vi "Set VI Reentrant Setting.vi"() -> ()   [LabVIEW 2016]
doc: "A wrapper engine for setting re-entrant setting for all VIs in a folder."
uses:
  <vilib>/Utility/error.llb/DialogType.ctl
  SLL Queued State Machine/Queue Driver/Create Queue.vi
  SLL Queued State Machine/Queue Driver/Enqueue an Item to Queue.vi
  SLL Queued State Machine/Queue Driver/Dequeue Queue.vi
  SLL Queued State Machine/Queue Driver/Enqueue N Items.vi
  SLL Queued State Machine/Queue Driver/Flush Queue.vi
  SLL Queued State Machine/Queue Driver/Release Queue.vi
  <vilib>/regexp/Match Regular Expression.xnode
  SLL Queued State Machine/SLL QSM.lvlib
panel:
  out "Progress":i32(slide) scale=0.0..10.0
  in  "VI Exclude Pattern":string="LV2"
  in  "Reentrancy Type":T1(ring)
  in  "Is Reentrant?":bool=TRUE
  in  "Folder Path":path
  out "Status":string
  in  "Run":bool
  # "Set VI Reentrant Setting"
  # "Sets the configured re-entrant settings for the VIs in the folder"
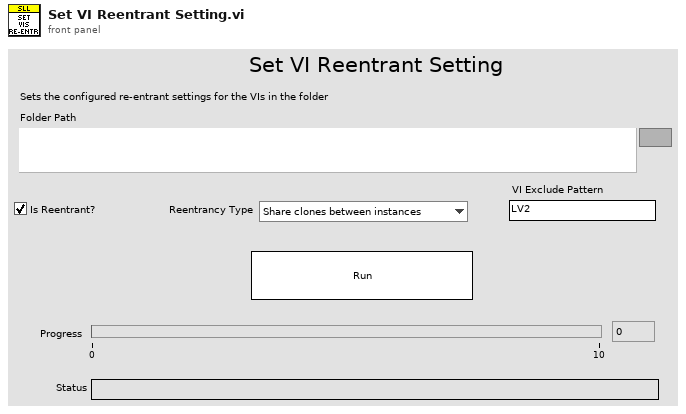
[diagram p1: front panel]
types:
  T1 = enum16{"Share clones between instances", "Preallocate clone for each instance"}
  T2 = enum32{"invalid VI type", "Standard VI", "Control VI", "Global VI", "Polymorphic VI", "Configuration VI", "SubSystem", "Facade VI", "Method VI", "Statechart Diagram VI"}
  T3 = typedef "DialogType.ctl" = u16
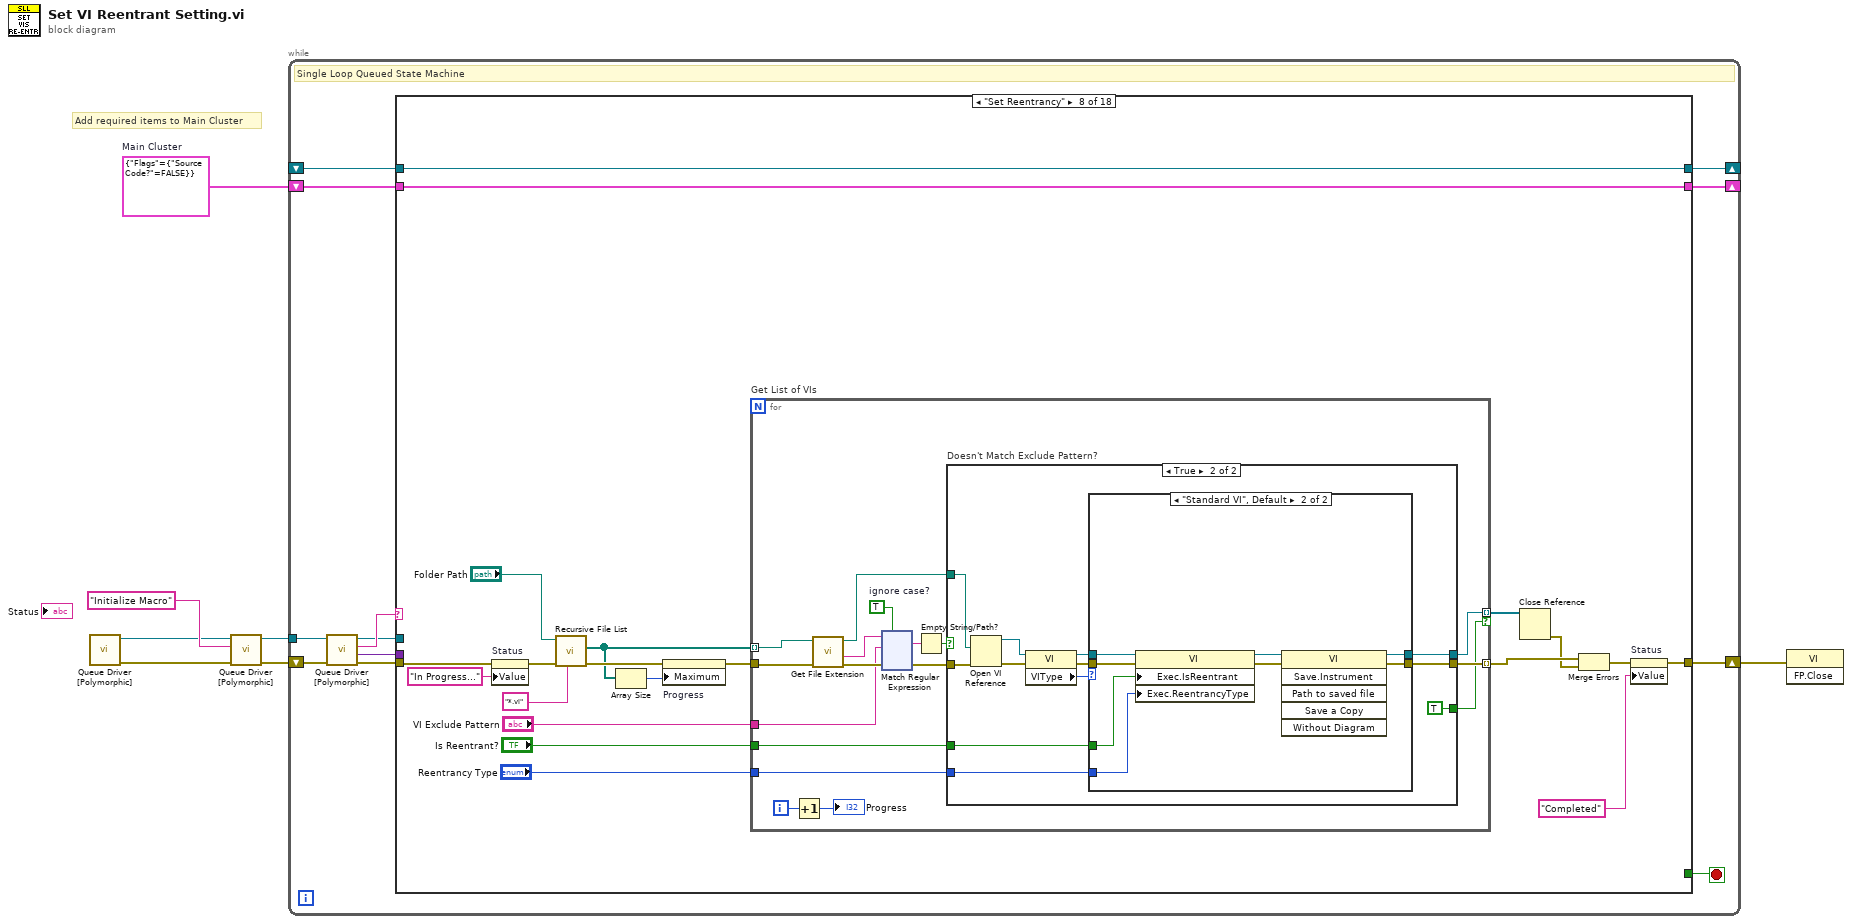
[diagram p0: block diagram]
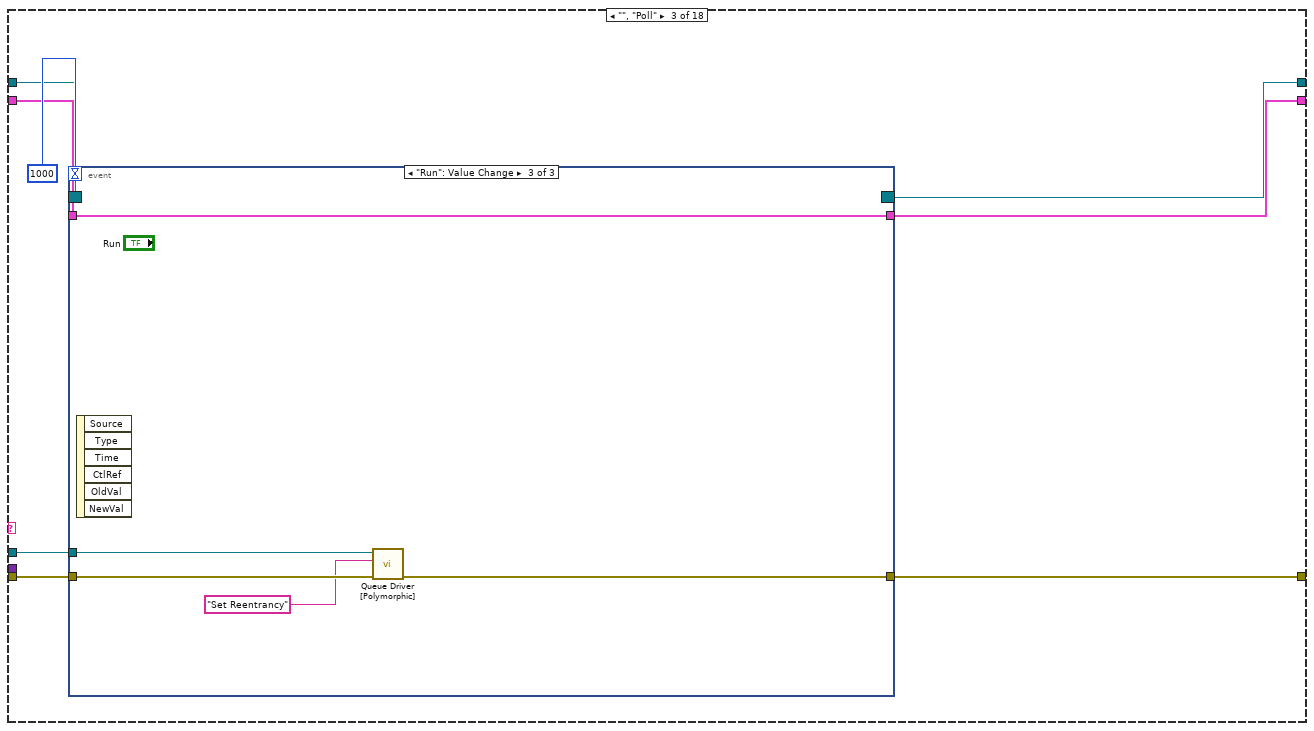
[diagram p4: hidden frame]
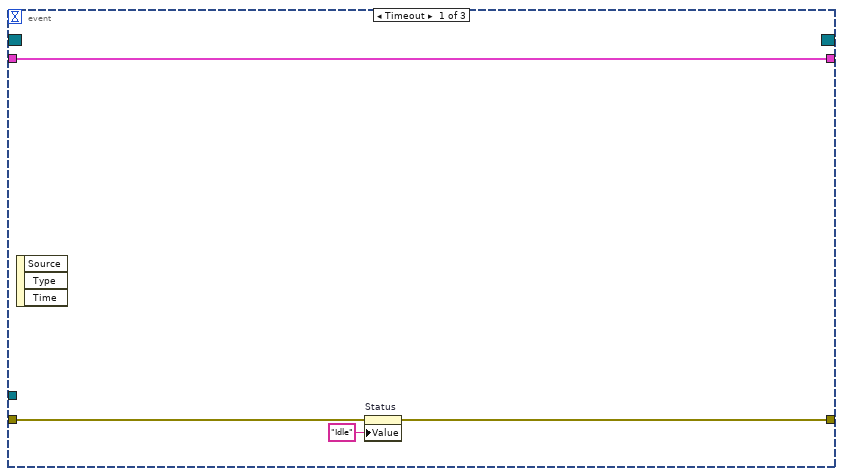
[diagram p5: hidden frame]
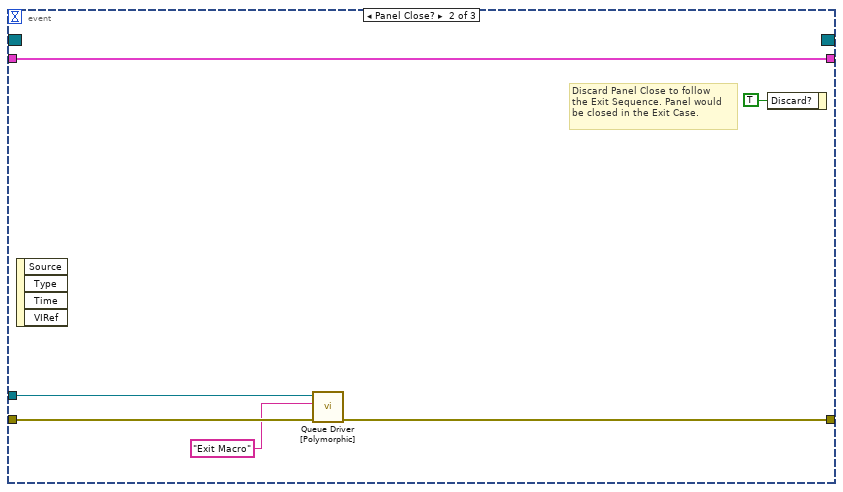
[diagram p6: hidden frame]
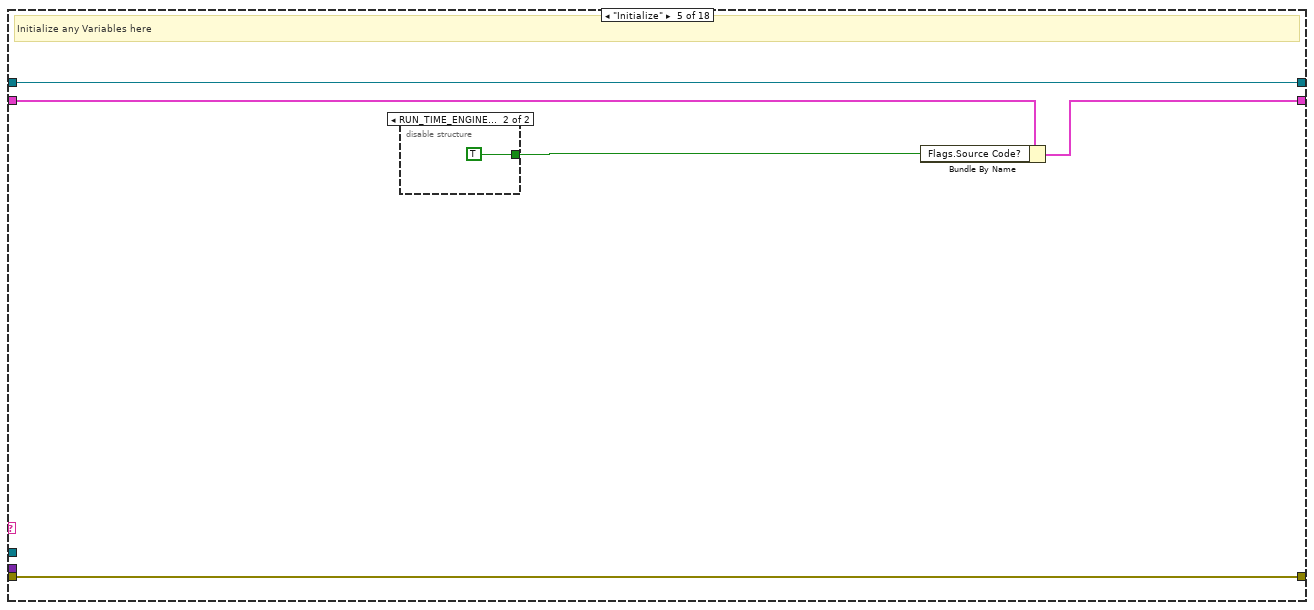
[diagram p8: hidden frame]
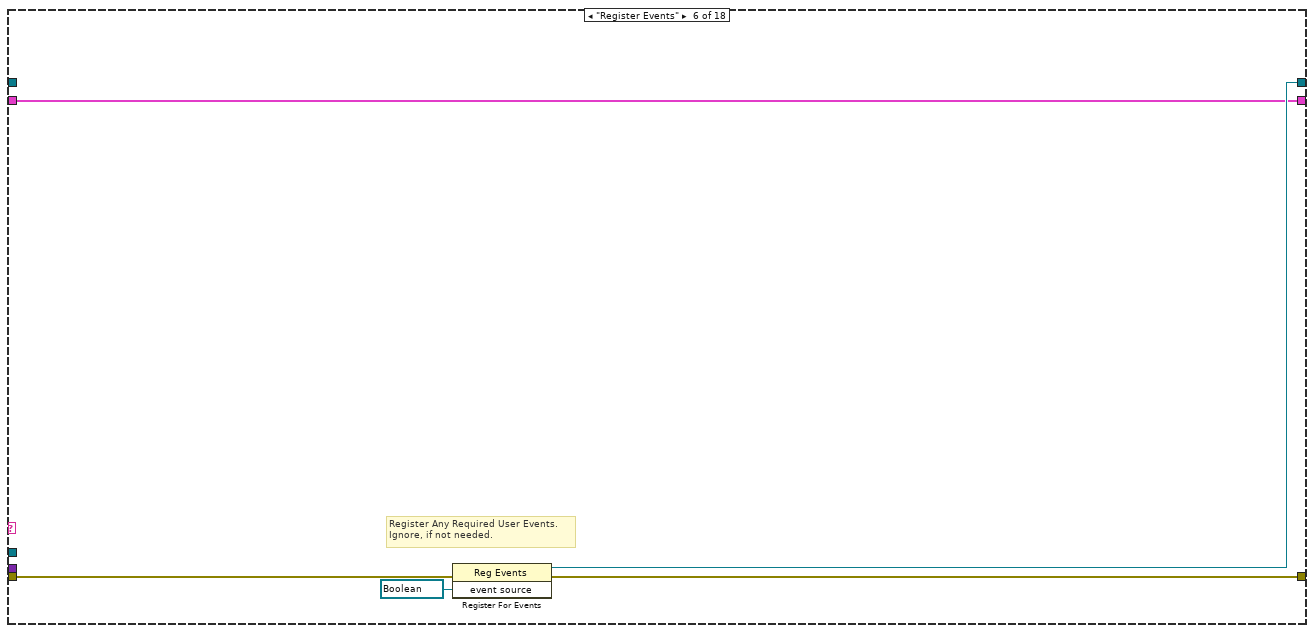
[diagram p10: hidden frame]
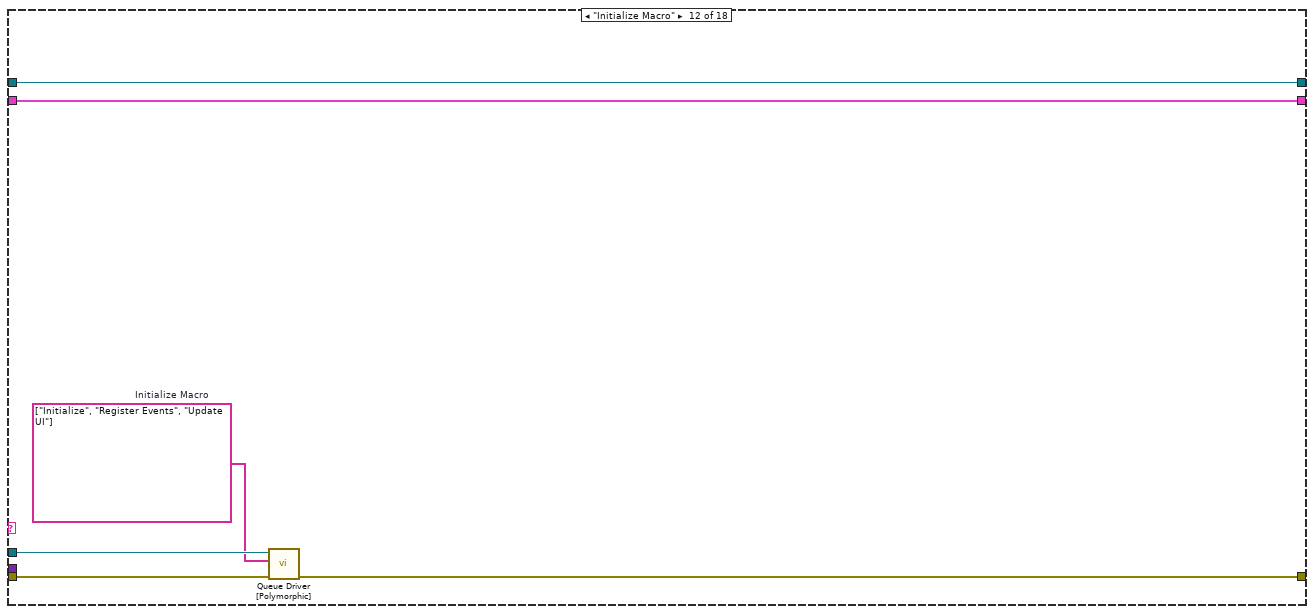
[diagram p17: hidden frame]
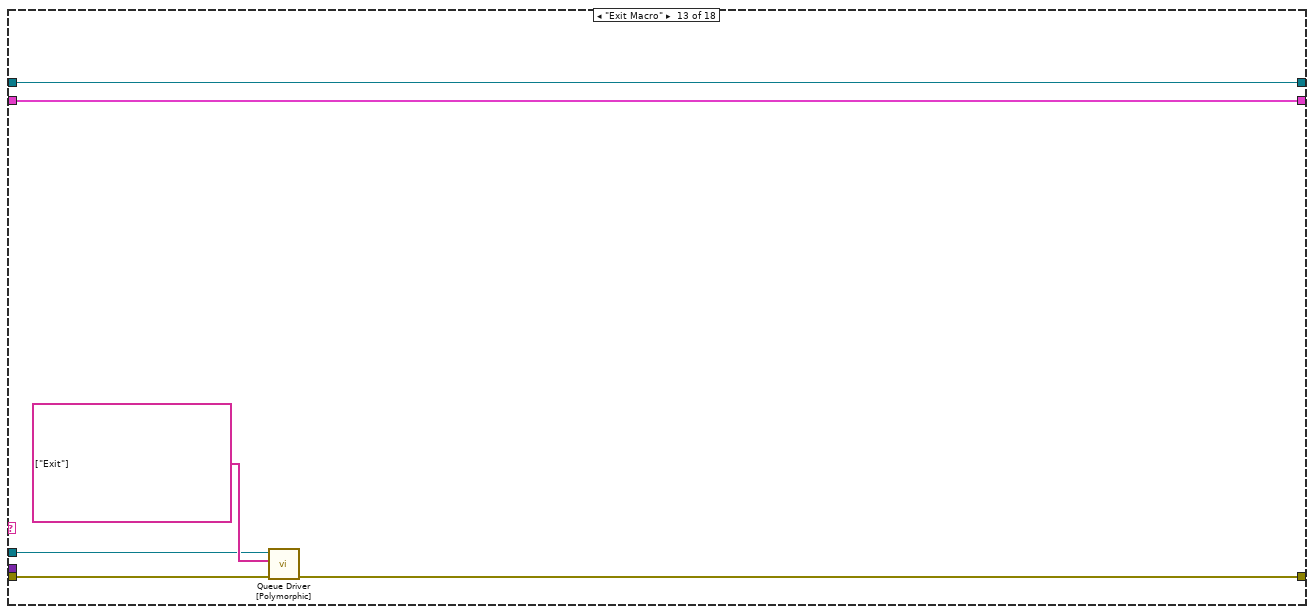
[diagram p18: hidden frame]
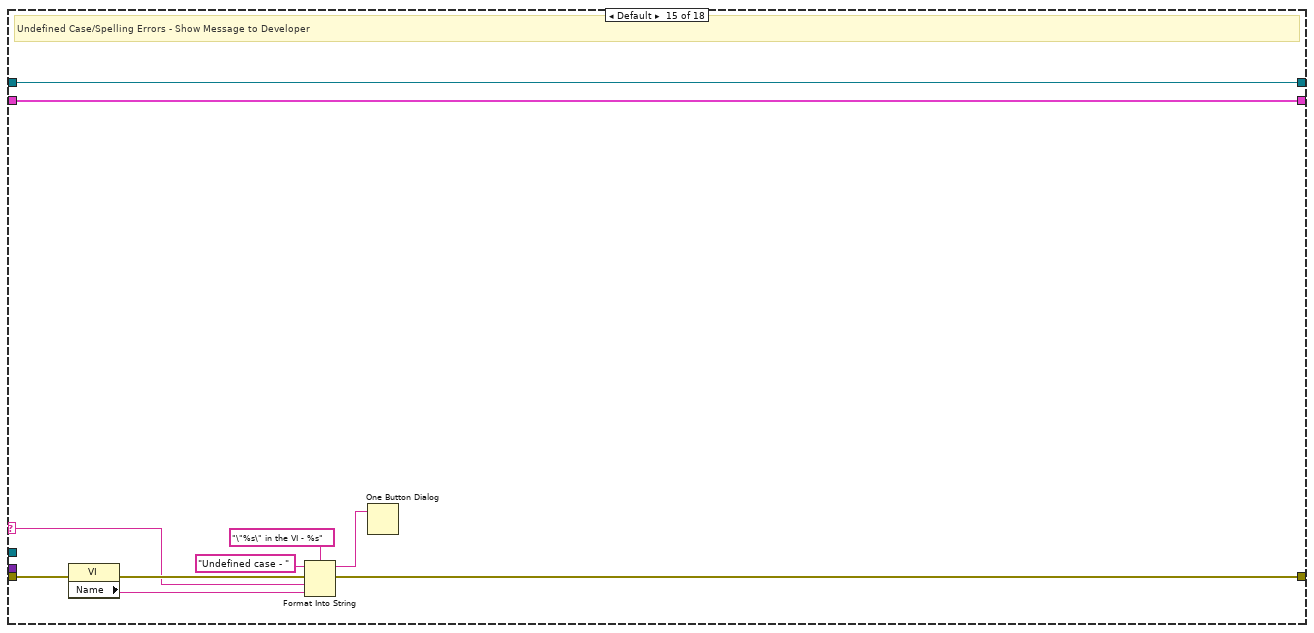
[diagram p20: hidden frame]
diagram:
  w5 = cluster{"Flags":cluster{"Source Code?":bool}} {"Flags"={"Source Code?"=FALSE}}  # Main Cluster
  # "Add required items to Main Cluster"
  n1 = call-poly "Queue Driver [Polymorphic].vi"() -> ("Error Out"=w7:errorcluster, "Queue Ref"=w3:refnum<queue>)  [unwired: 10 in]
  n2 = call-poly "Queue Driver [Polymorphic].vi"("Error In"=w7, "Item to Add"="Initialize Macro", "Queue Ref In"=w3) -> ("Error Out"=w6:errorcluster, "Queue Ref Out"=w2:refnum<queue>)  [unwired: 7 in]
  n3 = while "SLL Queued State Machine" {
    shift-right: [w17] -> w1
    shift-left: w6 -> [w19]
    shift-right: [w15] -> _
    shift-left: _ -> [w14]
    shift-right: [w13] -> _
    shift-left: w5 -> [w12]
    tunnel: w2 -> [w10]
    stop <- w16 stop-if-true
    # "Single Loop Queued State Machine"
    n4 = call-poly "Queue Driver [Polymorphic].vi"("Error In"=w19, "Queue Ref In"=w10) -> ("Error Out"=w18:errorcluster, "Data"=w8:variant, "Dequeue"=w11:string, "Queue Ref Out"=w9:refnum<queue>)  [unwired: 6 in]
    n5 = case "QSM Case Structure" shown="\"Set Reentrancy\"" w11 {
      selector: w11 -> [_ _ _ _ _ _ _ _ _ _ _ _ _ _ w264 _ _ _]
      tunnel: w18 -> [w22 w25 w31 w51 w56 w62 w65 w80 w242 w245 w248 w252 w258 w263 w267 w279 w282 w295]
      tunnel: [w22 w25 w32 w51 w56 w61 w65 w82 w242 w245 w248 w251 w257 w263 w270 w277 w282 w291] -> w17
      tunnel: [_ _ _ _ _ _ _ _ _ _ _ _ _ _ _ _ _ TRUE] -> w16
      tunnel: [w21 w24 w30 w50 w55 w60 w64 w85 w241 w244 w247 w254 w260 w262 w273 w276 w281 w294] -> w15
      tunnel: w14 -> [w21 w24 w29 w50 w55 _ w64 w85 w241 w244 w247 w254 w260 w262 w273 w276 w281 w294]
      tunnel: [w20 w23 w27 w49 w52 w59 w63 w84 w240 w243 w246 w253 w259 w261 w272 w275 w280 w293] -> w13
      tunnel: w12 -> [w20 w23 w28 w49 w53 w59 w63 w84 w240 w243 w246 w253 w259 w261 w272 w275 w280 w293]
      tunnel: w9 -> [_ _ w26 _ _ _ _ _ _ _ _ w250 w255 _ _ _ _ w284]
      tunnel: w8 -> [_ _ _ _ _ _ _ _ _ _ _ _ _ _ _ _ _ _]
      frame "/--------------- Read Me -----------------/" {
        # "General Purpose Queue Based State Machine for Any Use Case (main application, module, pop up message etc)\n\nAdvantages:\n1. No Need to Pass Queue References between Queue Driver VIs.\n2. This template can be safely used in multiple parallel running modules without any issues.\n3. This template can also be safely used even in cases where the VI is configured to be a Clone, where multiple \ninstances of the VI could be executing concurrently.\n\nHow to Use:\n1. Add necessary items to the Main Cluster.\n2. Use the Polymorphic Queue Driver for doing any queue operations. There is no need to pass the queue driver\nreference, as the Queue Driver automatically infers the reference based on the VI instance from which it is called.\n3. Add any required user events in the \"Register Events\" case. Ignore if not needed.\n4. Use \"Sequences\" section for defining any list of state calls, which could be used in multiple places. \nEg: Initialize Sequence, might be needed if we need to any reinitialization."
      }
      frame "/------------------ Poll -------------------/" {
      }
      frame "", "Poll" {
        n6 = event shown="[2] \"Run\": Value Change" {
          selector: w29 -> [_ _ _]
          dyn-events: [_ _ _] -> w30
          timeout: 1000 -> [_ _ _]
          tunnel: [w34 w42 w47] -> w32
          tunnel: w31 -> [w35 w43 w48]
          tunnel: w28 -> [w37 w41 w46]
          tunnel: [w37 w41 w46] -> w27
          tunnel: w26 -> [_ w38 w45]
          event Timeout {
            n7 = event-data() -> ()  [unwired: 1 in, 3 out]
            n8 = property on="Status" class="Str"(error in=w35, "Value"="Idle" ("Status")) -> (error out=w34:errorcluster)  [unwired: 1 in, 1 out]
          }
          event Panel Close? {
            # "Discard Panel Close to follow\nthe Exit Sequence. Panel would\nbe closed in the Exit Case."
            n9 = event-data() -> ()  [unwired: 1 in, 4 out]
            n10 = call-poly "Queue Driver [Polymorphic].vi"("Error In"=w43, "Item to Add"="Exit Macro" ("Enqueue"), "Queue Ref In"=w38) -> ("Error Out"=w42:errorcluster)  [unwired: 7 in, 1 out]
            n11 = event-data("Discard?"=TRUE) -> ()  [unwired: 1 in, 1 out]
          }
          event "Run": Value Change {
            n12 = event-data() -> ()  [unwired: 1 in, 6 out]
            n13 = call-poly "Queue Driver [Polymorphic].vi"("Error In"=w48, "Item to Add"="Set Reentrancy", "Queue Ref In"=w45) -> ("Error Out"=w47:errorcluster)  [unwired: 7 in, 1 out]
          }
        }
      }
      frame "/--------------- Initialize -----------------/" {
      }
      frame "Initialize" {
        # "Initialize any Variables here"
        n14 = disable-structure shown="RUN_TIME_ENGINE==False" {
          disable-tunnel: [_ TRUE] -> w54
          frame condition #0 {
          }
          frame condition #1 (active) {
          }
        }
        n15 = Bundle By Name(cluster=w53, "Flags.Source Code?"=w54) -> (w52:cluster{"Flags":cluster{"Source Code?":bool}})
      }
      frame "Register Events" {
        # "Register Any Required User Events. \nIgnore, if not needed."
        n16 = register-events(error in=w62, refnum<vi> refnum ("event source")) -> (reference out=w60:refnum<event-registration>, error out=w61:errorcluster)  [unwired: 1 in]
      }
      frame "/---------- Custom Case Splitter ----------/" {
      }
      frame "Set Reentrancy" {
        n17 = property on="Status" class="Str"(error in=w80, "Value"="In Progress..." ("Status")) -> (error out=w75:errorcluster)  [unwired: 1 in, 1 out]
        n18 = call <vilib>:"Recursive File List.vi"("pattern"="*.vi", "error in (no error)"=w75, "Folder Path"="Folder Path") -> ("error out"=w69:errorcluster, "All Files in Dir"=w67:path[])  [unwired: 4 in, 3 out]
        n19 = Array Size(array=w67) -> (size(s)=w66:i32)
        n20 = property on="Progress" class="Slide (strict)"(error in=w69, "Maximum"=w66) -> (error out=w68:errorcluster)  [unwired: 1 in, 1 out]
        n21 = for "Get List of VIs" {
          tunnel: [w102] -> w79 mode=indexing if=w91
          tunnel: w67 -> [w99] mode=indexing
          tunnel: w68 -> [w100]
          tunnel: [w101] -> w77 mode=indexing
          tunnel: "Is Reentrant?" -> [w90]
          tunnel: "Reentrancy Type" -> [w89]
          tunnel: "VI Exclude Pattern" -> [w88]
          i -> [w87]
          w95 = TRUE  # ignore case?
          n22 = Increment(x=w87) -> (x+1=→"Progress":i32)
          n23 = call <vilib>:"Get File Extension.vi"("error in (no error)"=w100, "file"=w99) -> ("error out"=w97:errorcluster, "filename without extension"=w94:string, "dup file"=w98:path)  [unwired: 5 in, 2 out]
          n24 = xnode "Match Regular Expression"("input string"=w94, "regular expression"=w88, "error in"=w97, "ignore case? (F)"=w95) -> ("whole match"=w93:string, "error out"=w96:errorcluster)  [unwired: 2 in, 3 out]
          n25 = Empty String/Path?(string/path=w93) -> (empty?=w92:bool)
          n26 = case "Doesn't Match Exclude Pattern?" shown="True" w92 {
            tunnel: [_ w115] -> w102
            tunnel: [w103 w114] -> w101
            tunnel: w98 -> [_ w113]
            tunnel: w96 -> [w103 w112]
            tunnel: [_ TRUE] -> w91
            tunnel: w90 -> [_ w105]
            tunnel: w89 -> [_ w104]
            frame False {
            }
            frame True {
              n27 = Open VI Reference(vi path=w113, error in (no error)=w112) -> (vi reference=w110:refnum<vi>, error out=w111:errorcluster)  [unwired: 4 in]
              n28 = property class="VI"(reference=w110, error in=w111) -> (reference out=w109:refnum<vi>, error out=w108:errorcluster, "VIType"=w107:T2)
              n29 = case shown="\"Standard VI\", Default" w107 {
                tunnel: [w116 w123] -> w115
                tunnel: [w117 w122] -> w114
                tunnel: w109 -> [w116 w121]
                tunnel: w108 -> [w117 w120]
                tunnel: w105 -> [_ w119]
                tunnel: w104 -> [_ w118]
                frame "Polymorphic VI" {
                  # "Note: Polymorphic VIs will result in error when setting the re-entrancy setting"
                  # "Ignoring for Polymorphic VIs"
                }
                frame "Standard VI", Default {
                  n30 = property class="VI"(reference=w121, error in=w120, "Exec.IsReentrant"=w119, "Exec.ReentrancyType"=w118) -> (reference out=w124:refnum<vi>, error out=w125:errorcluster)
                  n31 = invoke class="VI" method="Save.Instrument"(reference=w124, error in=w125) -> (reference out=w123:refnum<vi>, error out=w122:errorcluster)  [unwired: 4 in, 4 out]
                }
              }
            }
          }
        }
        n32 = Close Reference(reference=w79) -> (error out=w76:errorcluster)  [unwired: 1 in]
        n33 = Merge Errors(w77, w76) -> (w74:errorcluster)
        n34 = property on="Status" class="Str"(error in=w74, "Value"="Completed" ("Status")) -> (error out=w82:errorcluster)  [unwired: 1 in, 1 out]
      }
      frame "/-------------- User Interface --------------/" {
        # "Duplicate this case to create additional case splitters for readability"
      }
      frame "Update UI" {
        # "Update Front Panel Controls in this Case"
      }
      frame "/----------------- Macros -----------------/" {
      }
      frame "Initialize Macro" {
        w249 = string[] ["Initialize", "Register Events", "Update UI"]  # Initialize Macro
        n35 = call-poly "Queue Driver [Polymorphic].vi"("Error In"=w252, "Enqueue N"=w249, "Queue Ref In"=w250) -> ("Error Out"=w251:errorcluster)  [unwired: 7 in, 1 out]
      }
      frame "Exit Macro" {
        n36 = call-poly "Queue Driver [Polymorphic].vi"("Error In"=w258, "Enqueue N"=string[] ["Exit"], "Queue Ref In"=w255) -> ("Error Out"=w257:errorcluster)  [unwired: 7 in, 1 out]
      }
      frame "/-------------- Error Handler--------------/" {
      }
      frame Default {
        # "Undefined Case/Spelling Errors - Show Message to Developer"
        n37 = property class="VI"(error in=w267) -> (error out=w266:errorcluster, "Name"=w265:string)  [unwired: 1 in, 1 out]
        n38 = Format Into String(format string="\"%s\" in the VI - %s" ("message"), initial string="Undefined case - ", error in=w266, w264, w265) -> (resulting string=w268:string, error out=w270:errorcluster)
        n39 = One Button Dialog(message=w268) -> ()  [unwired: 1 in, 1 out]
      }
      frame "Error" {
        w274 = T3 2 items=["no dialog", "OK message", "continue or stop message", "OK message + warnings", "continue/stop + warnings"] ("type of dialog (OK msg:1)")
        # "Handle the Error"
        n40 = call <vilib>:"Simple Error Handler.vi"("type of dialog (OK msg:1)"=w274, "error in (no error)"=w279) -> ("error out"=w278:errorcluster)  [unwired: 3 in, 4 out]
        n41 = call <vilib>:"Clear Errors.vi"("error in (no error)"=w278) -> ("error out"=w277:errorcluster)  [unwired: 5 in, 1 out]
      }
      frame "/------------------- Exit --------------------/" {
      }
      frame "Exit" {
        n42 = call-poly "Queue Driver [Polymorphic].vi"("Error In"=w295, "Queue Ref In"=w284) -> ("Error Out"=w296:errorcluster, "Queue Ref Out"=w283:refnum<queue>)  [unwired: 7 in, 1 out]
        n43 = Unbundle By Name(w293) -> ("Flags.Source Code?"=w286:bool)
        n44 = call-poly "Queue Driver [Polymorphic].vi"("Error In"=w296, "Queue Ref In"=w283) -> ("Error Out"=w292:errorcluster)  [unwired: 9 in]
        n45 = Call Chain() -> (call chain=w290:string[])
        n46 = Array Size(array=w290) -> (size(s)=w289:i32)
        n47 = Equal?(x=w289, y=1) -> (x = y?=w287:bool)
        n48 = And(x=w286, y=w287) -> (x .and. y?=w285:bool)
        n49 = case "Skip Panel Close when in Source\nCode and is the top most caller" shown="True" w285 {
          tunnel: w292 -> [w299 w301]
          tunnel: [w300 w301] -> w291
          frame False {
            # "Close Panel"
            n50 = invoke class="VI" method="FP.Close"() -> (error out=w298:errorcluster)  [unwired: 3 in, 2 out]
            n51 = Merge Errors(w299, w298) -> (w300:errorcluster)
          }
          frame True {
            # "Do Not Close Panel"
          }
        }
      }
    }
  }
  n52 = invoke class="VI" method="FP.Close"(error in=w1) -> ()  [unwired: 2 in, 3 out]
